vi "LDC-37X4C Set TEC Temperature Limit.vi"(8 "error in (no error)":errorcluster, 10 "Limit":dbl min=-100.0 max=199.9 step=0.1, 11 "VISA resource name":refnum<visa-resource-name>) -> (0 "error out":errorcluster, 3 "VISA resource name out":refnum<visa-resource-name>)   [LabVIEW 2021]
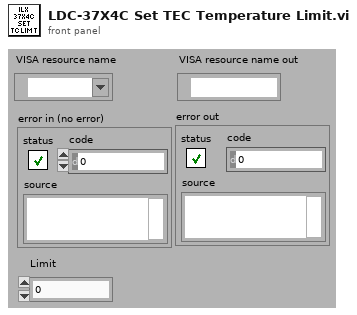
[diagram p1: front panel]
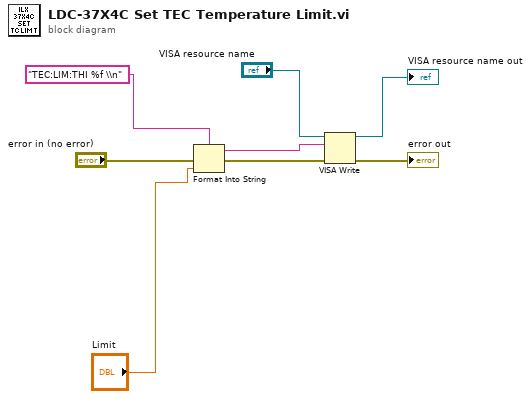
[diagram p0: block diagram]
diagram:
  n1 = Format Into String(format string="TEC:LIM:THI %f \\n", error in="error in (no error)", "Limit") -> (resulting string=w7:string, error out=w5:errorcluster)  [unwired: 1 in]
  n2 = VISA Write(VISA resource name="VISA resource name", write buffer=w7, error in (no error)=w5) -> (VISA resource name out=→"VISA resource name out":refnum<visa-resource-name>, error out=→"error out":errorcluster)  [unwired: 1 out]
